vi "ExecASYNCs.vi"(9 "messageIn":string, 11 "nameValueArray":cluster{"String":string, "Setpoint":dbl}[](array[cluster])) -> (1 "messageOut":string)   [LabVIEW 2021]
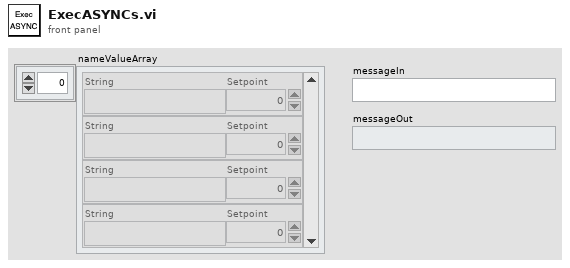
[diagram p1: front panel]
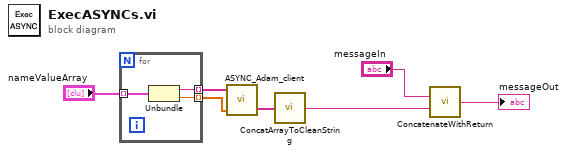
[diagram p0: block diagram]
diagram:
  n1 = for {
    tunnel: "nameValueArray" -> [w10] mode=indexing
    tunnel: [w9] -> w2 mode=indexing
    tunnel: [w8] -> w3 mode=indexing
    n2 = Unbundle(w10) -> ("String"=w9:string, "Setpoint"=w8:dbl)
  }
  n3 = call "ASYNC_Adam_client.vi"("Values"=w3, "Channel Names"=w2) -> ("Scan Comments"=w4:string[])  [unwired: 1 in, 1 out]
  n4 = call "ConcatArrayToCleanString.vi"("stringArray"=w4) -> ("cleanDelimitedString"=w6:string)  [unwired: 1 in]
  n5 = call "ConcatenateWithReturn.vi"("baseString"="messageIn", "additionalString"=w6) -> ("outputString"=→"messageOut":string)  [unwired: 13 in]
